vi "PSCMD_Toolbar Command.vi"(8 "error in (no error)":errorcluster, 10 "Data":variant, 11 "Command":T1) -> (0 "error out":errorcluster)   [LabVIEW 2016]
uses:
  Controls/PSDAQEG_Commoand Type.ctl
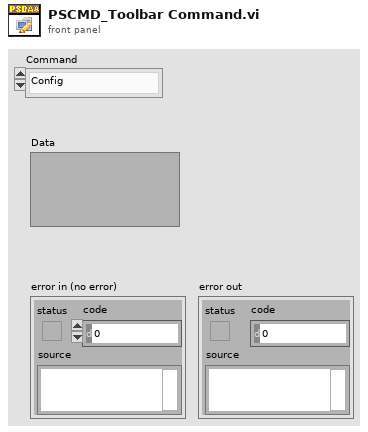
[diagram p1: front panel]
types:
  T1 = typedef "PSDAQEG_Commoand Type.ctl" = enum16{"Config", "Run", "Pause", "Stop", "Save", "Connect"}
  T2 = cluster{"Main Queue":string, "DAQ Queue":string, "ANA Queue":string, "CUI Queue":string, "Q-FocusList":string, "Q-Toolbar":string, "Q-Config":string}
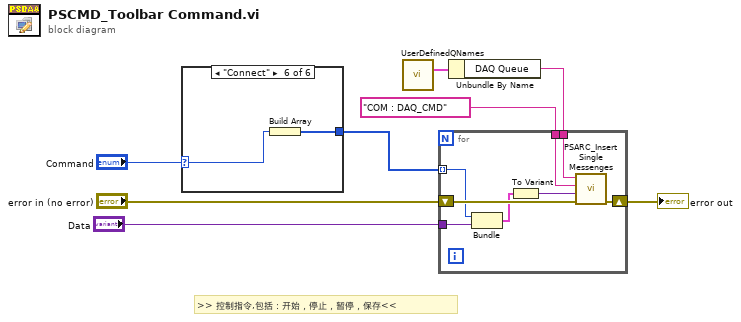
[diagram p0: block diagram]
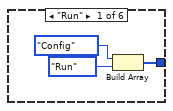
[diagram p2: hidden frame]
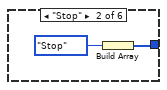
[diagram p3: hidden frame]
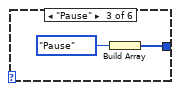
[diagram p4: hidden frame]
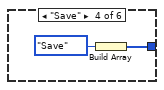
[diagram p5: hidden frame]
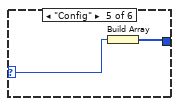
[diagram p6: hidden frame]
diagram:
  # ">> 控制指令,包括：开始，停止，暂停，保存<<"
  n1 = case shown="\"Connect\"" "Command" {
    selector: "Command" -> [_ _ _ _ w18 w20]
    tunnel: [w11 w13 w15 w17 w19 w21] -> w8
    frame "Run" {
      n2 = Build Array(PSDAQEG_Commoand_Type."Config" ("Command"), PSDAQEG_Commoand_Type."Run" ("Command")) -> (w11:T1[])
    }
    frame "Stop" {
      n3 = Build Array(PSDAQEG_Commoand_Type."Stop" ("Command")) -> (w13:T1[])
    }
    frame "Pause" {
      n4 = Build Array(PSDAQEG_Commoand_Type."Pause" ("Command")) -> (w15:T1[])
    }
    frame "Save" {
      n5 = Build Array(PSDAQEG_Commoand_Type."Save" ("Command")) -> (w17:T1[])
    }
    frame "Config" {
      n6 = Build Array(w18) -> (w19:T1[])
    }
    frame "Connect" {
      n7 = Build Array(w20) -> (w21:T1[])
    }
  }
  n8 = call "UserDefinedQNames.vi"() -> ("All Queues"=w2:T2)  [unwired: 11 in]
  n9 = Unbundle By Name(w2) -> ("DAQ Queue"=w1:string)
  n10 = for {
    tunnel: "COM : DAQ_CMD" -> [w27]
    tunnel: w1 -> [w26]
    shift-right: [w28] -> w4
    shift-left: "error in (no error)" -> [w29]
    tunnel: w8 -> [w23] mode=indexing
    tunnel: "Data" -> [w24]
    n11 = Bundle("Command"=w23, "Data"=w24) -> (w22:cluster{"Command":T1, "Data":variant})  [unwired: 1 in]
    n12 = To Variant(anything=w22) -> (Variant=w25:variant)
    n13 = call <vilib>:"PSARC_Insert Single Messenges.vi"("error in (no error)"=w29, "Data"=w25, "Order"=w27, "Queue Name"=w26) -> ("error out"=w28:errorcluster)  [unwired: 7 in]
  }
  "error out" <- w4
